vi "Get Chamber Status-UTF-Teardown.vi"   [LabVIEW 2018]
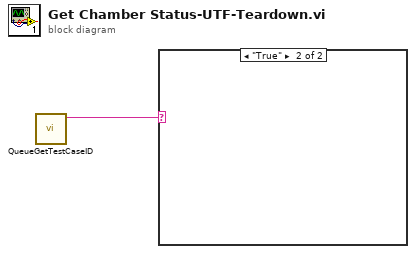
[diagram p0: block diagram]
diagram:
  n1 = call "QueueGetTestCaseID.vi"() -> ("test case ID"=w1:string)  [unwired: 11 in]
  n2 = case shown="\"True\"" w1 {
    frame "False", Default {
    }
    frame "True" {
    }
  }
